vi "CheckEquilibrium.vi"(8 "error in (no error)":errorcluster, 9 "Eventually replace this with output from an algorithm to check equilibrium":bool, 10 "queue in":refnum<queue>, 11 "Data Cluster":T1={"Current DoE"=[], "SSI 1 Flow Rate"=0.0, "SSI 2 Flow Rate"=0.0, "FLOM 1 Flow Rate"=0.0, "FLOM 2 Flow Rate"=0.0, "Pumps Running?"=FALSE, "Boolean 2"=FALSE, "Boolean 3"=FALSE, "Boolean 4"=FALSE, "At Equilibrium?"=FALSE, "Script Running?"=FALSE, "Current Script Iteration"=0.0, "Total Script Iterations"=0.0, "FLOM Pumps VISA"="COM2", "SSI 1 Pump VISA"="COM76", "SSI 2 Pump VISA"="COM74", "Huber Unistat VISA"="COM1", "SSI 3 Pump VISA"="COM76", "SSI 4 Pump VISA"="COM76", "SSI 4 Flow Rate"=0.0, "SSI 3 Flow Rate"=0.0, "Flow Meter 1"="COM76", "Flow Meter 2"="COM76", "Flow Meter 3"="COM76", "Flow Meter 4"="COM76", "Flow Meter 1 Rate "=0.0, "Flow Meter 2 Rate"=0.0, "Flow Meter 3 Rate"=0.0, "Flow Meter 4 Rate"=0.0, "SSI 1 Flow Setpoint"=0.0, "SSI 2 Flow Setpoint"=0.0, "SSI 3 Flow Setpoint"=0.0, "SSI 4 Flow Setpoint"=0.0, "Temperature Setpoint"=0.0} {"Current DoE" format="%0.3f"}) -> (0 "error out":errorcluster, 2 "queue out":refnum<queue>, 3 "Data Cluster 2":T1={"Current DoE"=[], "SSI 1 Flow Rate"=0.0, "SSI 2 Flow Rate"=0.0, "FLOM 1 Flow Rate"=0.0, "FLOM 2 Flow Rate"=0.0, "Pumps Running?"=FALSE, "Boolean 2"=FALSE, "Boolean 3"=FALSE, "Boolean 4"=FALSE, "At Equilibrium?"=FALSE, "Script Running?"=FALSE, "Current Script Iteration"=0.0, "Total Script Iterations"=0.0, "FLOM Pumps VISA"="COM2", "SSI 1 Pump VISA"="COM76", "SSI 2 Pump VISA"="COM74", "Huber Unistat VISA"="COM1", "SSI 3 Pump VISA"="COM76", "SSI 4 Pump VISA"="COM76", "SSI 4 Flow Rate"=0.0, "SSI 3 Flow Rate"=0.0, "Flow Meter 1"="COM76", "Flow Meter 2"="COM76", "Flow Meter 3"="COM76", "Flow Meter 4"="COM76", "Flow Meter 1 Rate "=0.0, "Flow Meter 2 Rate"=0.0, "Flow Meter 3 Rate"=0.0, "Flow Meter 4 Rate"=0.0, "SSI 1 Flow Setpoint"=0.0, "SSI 2 Flow Setpoint"=0.0, "SSI 3 Flow Setpoint"=0.0, "SSI 4 Flow Setpoint"=0.0, "Temperature Setpoint"=0.0} {"Current DoE" format="%0.3f"})   [LabVIEW 2015]
uses:
  --Controls and TypeDefs--/DoE_Control_Cluster.ctl
panel:
  # "VI to check P, T, and Chemical Equilibrium"
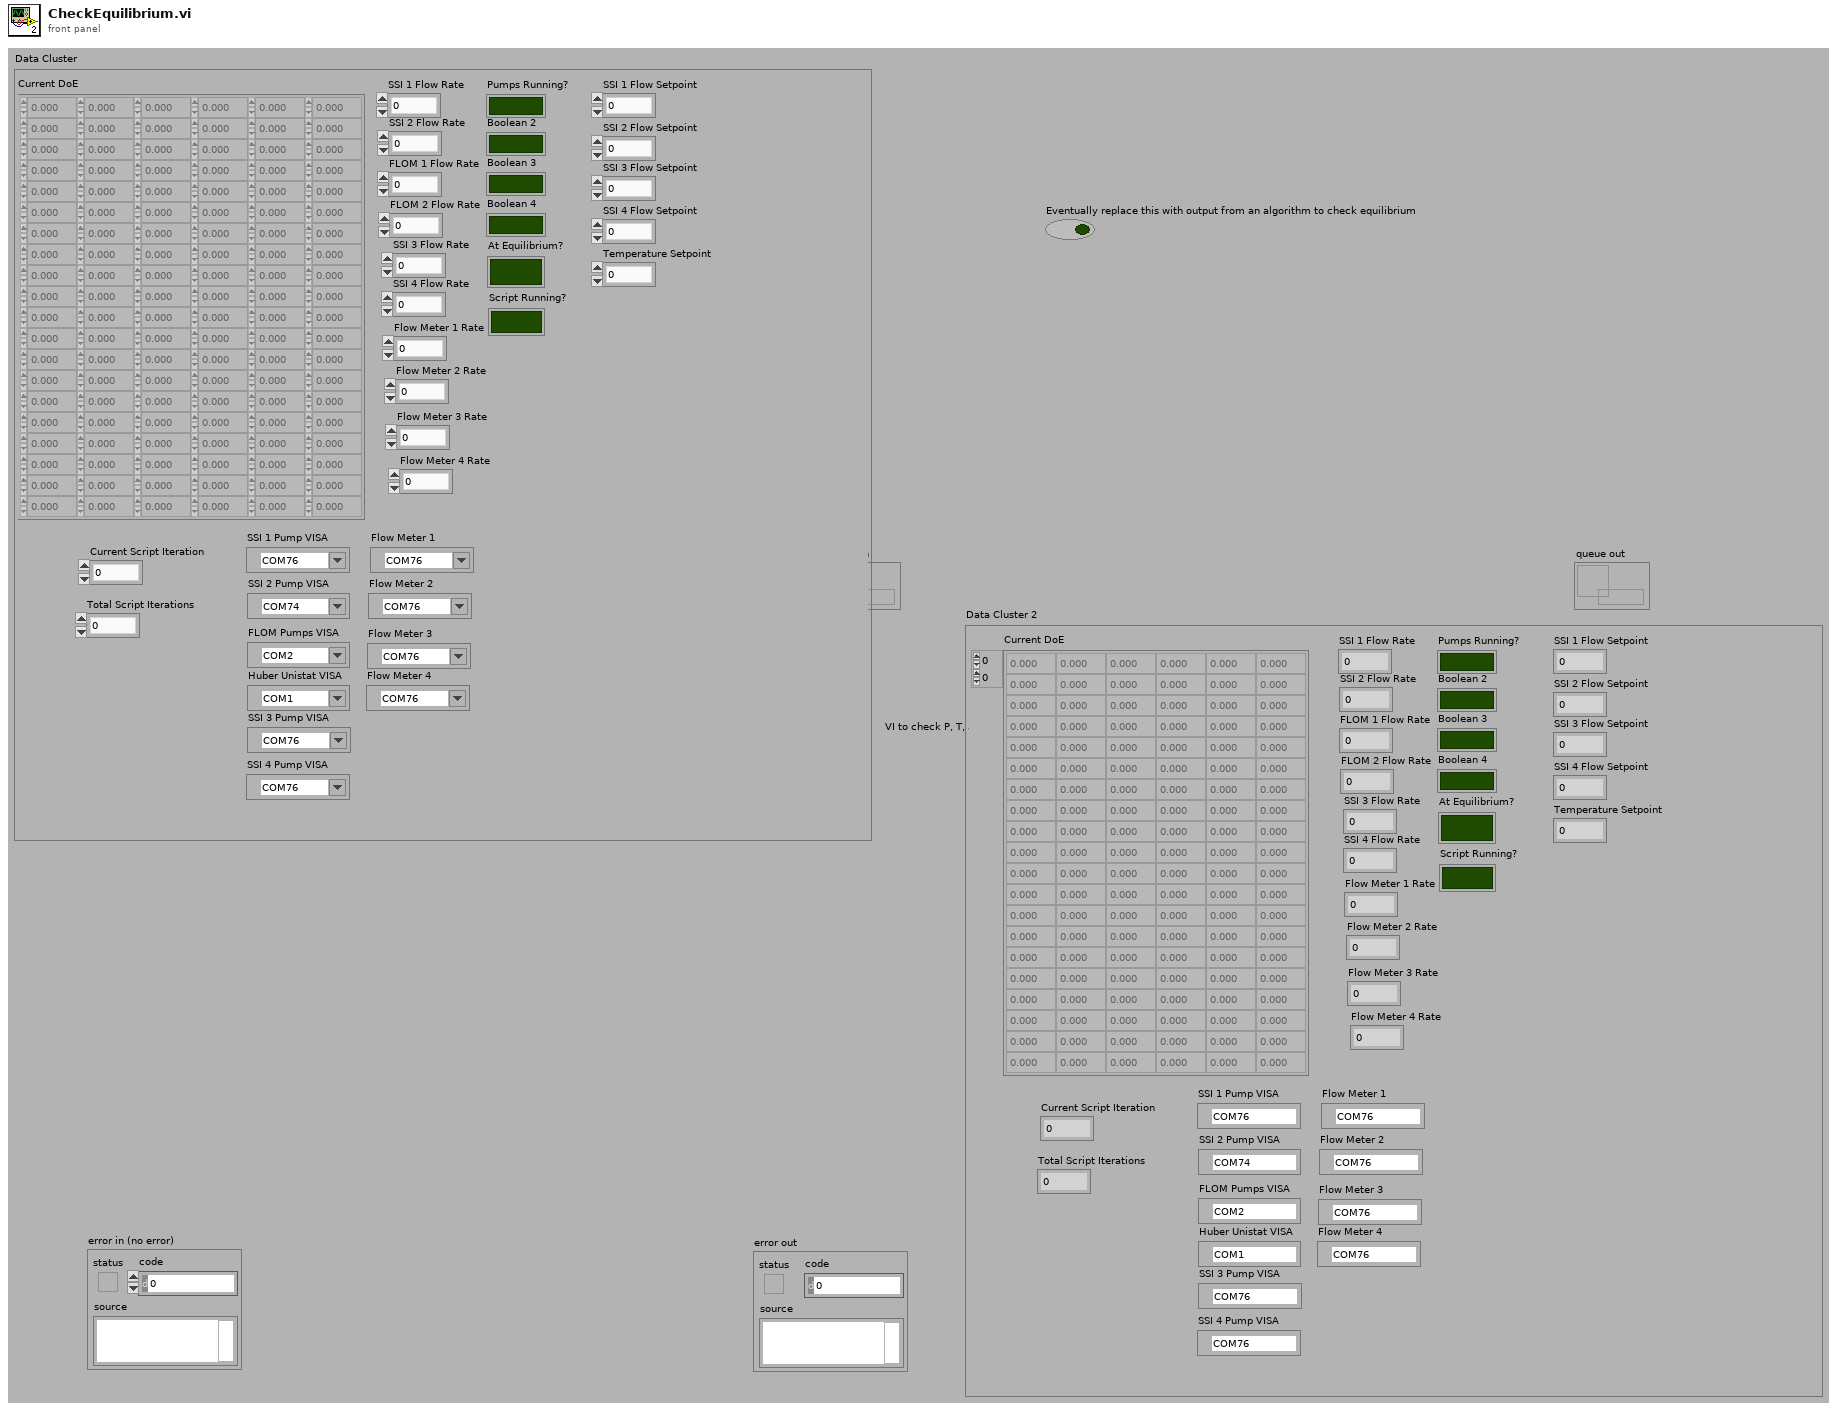
[diagram p1: front panel]
types:
  T1 = typedef "DoE_Control_Cluster.ctl" = cluster{"Current DoE":dbl[][], "SSI 1 Flow Rate":dbl, "SSI 2 Flow Rate":dbl, "FLOM 1 Flow Rate":dbl, "FLOM 2 Flow Rate":dbl, "Pumps Running?":bool, "Boolean 2":bool, "Boolean 3":bool, "Boolean 4":bool, "At Equilibrium?":bool, "Script Running?":bool, "Current Script Iteration":dbl, "Total Script Iterations":dbl, "FLOM Pumps VISA":refnum<visa-resource-name>, "SSI 1 Pump VISA":refnum<visa-resource-name>, "SSI 2 Pump VISA":refnum<visa-resource-name>, "Huber Unistat VISA":refnum<visa-resource-name>, "SSI 3 Pump VISA":refnum<visa-resource-name>, "SSI 4 Pump VISA":refnum<visa-resource-name>, "SSI 4 Flow Rate":dbl, "SSI 3 Flow Rate":dbl, "Flow Meter 1":refnum<visa-resource-name>, "Flow Meter 2":refnum<visa-resource-name>, "Flow Meter 3":refnum<visa-resource-name>, "Flow Meter 4":refnum<visa-resource-name>, "Flow Meter 1 Rate ":dbl, "Flow Meter 2 Rate":dbl, "Flow Meter 3 Rate":dbl, "Flow Meter 4 Rate":dbl, "SSI 1 Flow Setpoint":dbl, "SSI 2 Flow Setpoint":dbl, "SSI 3 Flow Setpoint":dbl, "SSI 4 Flow Setpoint":dbl, "Temperature Setpoint":dbl}
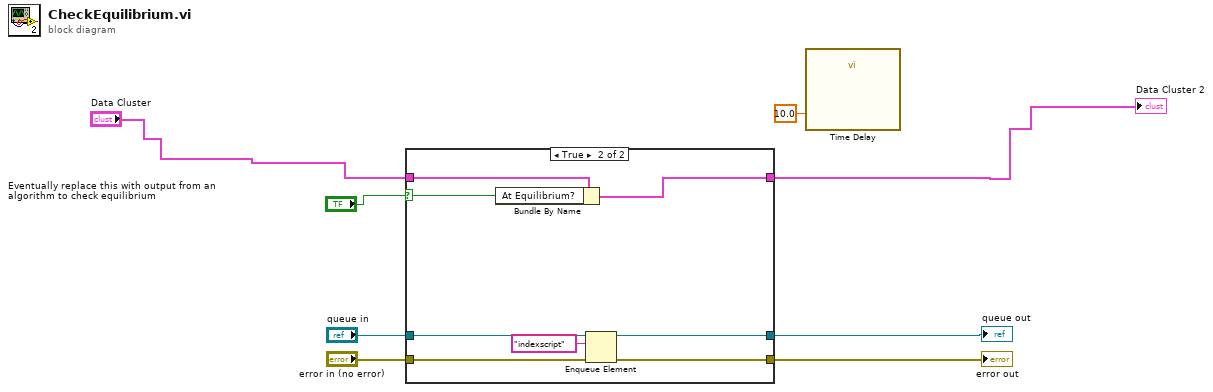
[diagram p0: block diagram]
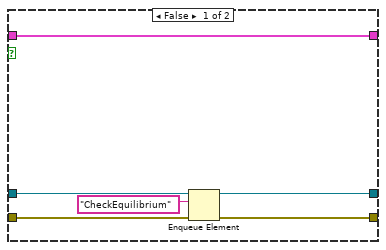
[diagram p2: hidden frame]
diagram:
  n1 = case shown="True" "Eventually replace this with output from an algorithm to check equilibrium" {
    selector: "Eventually replace this with output from an algorithm to check equilibrium" -> [_ w20]
    tunnel: "Data Cluster" -> [w14 w22]
    tunnel: [w14 w21] -> w1
    tunnel: "queue in" -> [w13 w19]
    tunnel: [w9 w17] -> w6
    tunnel: "error in (no error)" -> [w11 w16]
    tunnel: [w10 w15] -> w4
    frame False {
      n2 = Enqueue Element(queue=w13, element="CheckEquilibrium", error in (no error)=w11) -> (queue out=w9:refnum<queue>, error out=w10:errorcluster)  [unwired: 1 in, 1 out]
    }
    frame True {
      n3 = Bundle By Name(cluster=w22, "At Equilibrium?"=w20) -> (w21:T1)
      n4 = Enqueue Element(queue=w19, element="indexscript", error in (no error)=w16) -> (queue out=w17:refnum<queue>, error out=w15:errorcluster)  [unwired: 1 in, 1 out]
    }
  }
  "queue out" <- w6
  "error out" <- w4
  "Data Cluster 2" <- w1
  n5 = call "Time Delay"("Delay Time (s)"=10.0) -> ()  [unwired: 10 in, 1 out]
